vi "formula resolvente.vi"() -> ()   [LabVIEW 2018]
panel:
  out "x2":dbl
  out "x1":dbl
  in  "c":dbl
  in  "b":dbl
  in  "a":dbl
  # "Fórmula Resolvente"
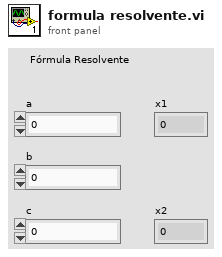
[diagram p1: front panel]
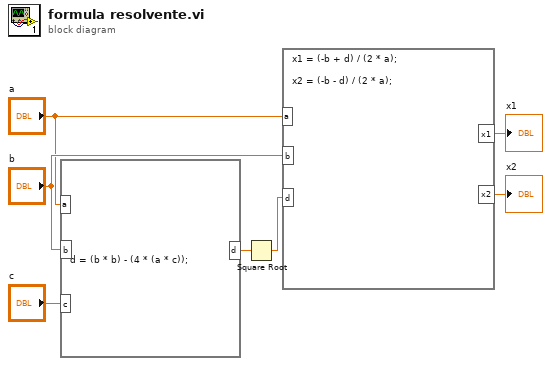
[diagram p0: block diagram]
diagram:
  n1 = formula code="d = (b * b) - (4 * (a * c));"("a"="a", "b"="b", "c"="c") -> ("d"=w6:dbl)
  n2 = Square Root(x=w6) -> (sqrt(x)=w5:dbl)
  n3 = formula code="x1 = (-b + d) / (2 * a);\n\nx2 = (-b - d) / (2 * a);"("a"="a", "b"="b", "d"=w5) -> ("x1"=→"x1":dbl, "x2"=→"x2":dbl)
